vi "UHR-Fleezers Control (host) -Leonardo 04-2018 V2.vi"(0 "Tab Control":T5(tab)=enum."Trap Control (RF)") -> ()   [LabVIEW 2013] (continued)
        n954 = event-data() -> ()  [unwired: 7 out]
        n955 = call "hamilton_controller.vi"("Open?"="Inject Bottom", "valve"=enum16{"A", "B", "C", "D", "ALL"}."C", "action"=T21."MOVE VALVE") -> ()  [unwired: 8 in, 1 out]
      }
      event "Shunt:": Value Change {
        n956 = event-data() -> ()  [unwired: 7 out]
        n957 = call "hamilton_controller.vi"("Open?"="Shunt:", "valve"=enum16{"A", "B", "C", "D", "ALL"}."D", "action"=T21."MOVE VALVE") -> ()  [unwired: 8 in, 1 out]
      }
      event "Flip Green Filter": Value Change {
        n958 = event-data() -> ()  [unwired: 7 out]
        n959 = local write "Flip Green Filter"("Flip Green Filter") -> ()
        n960 = flat-sequence {
          tunnel: w1540 -> [w1545]
          tunnel: w1539 -> [w1544]
          tunnel: [w1542] -> w1537
          tunnel: [w1541] -> w1536
          tunnel: [w1547] -> w1535
          tunnel: w1537 -> [w1547]
          tunnel: [w1546] -> w1534
          tunnel: w1536 -> [w1546]
          tunnel: w1535 -> [w1551]
          tunnel: w1534 -> [w1550]
          tunnel: [w1549] -> w1538
          frame #0 {
            n961 = xnode "Read/Write Control"("FPGA VI Reference In"=w1545, "error in"=w1544, "Green Filter Flipper"=TRUE) -> ("FPGA VI Reference Out"=w1542:T20, "error out"=w1541:errorcluster)
          }
          frame #1 {
            n962 = Wait (ms)(milliseconds to wait=u32 100) -> ()  [unwired: 1 out]
          }
          frame #2 {
            n963 = xnode "Read/Write Control"("FPGA VI Reference In"=w1551, "error in"=w1550, "Green Filter Flipper"=FALSE) -> ("error out"=w1549:errorcluster)  [unwired: 1 out]
          }
        }
      }
      event "Pump 1 contents", "Pump 3 contents": Value Change {
        n964 = event-data() -> ()  [unwired: 7 out]
        n965 = local read "Pump 1 contents"() -> (→"Pump 1 cont disp":string)
        n966 = local read "Pump 3 contents"() -> (→"Pump 3 cont disp":string)
      }
      event "Reset Trap Pos. FB": Value Change {
        n967 = event-data() -> ()  [unwired: 7 out]
        n968 = xnode "Read/Write Control"("FPGA VI Reference In"=w1557, "error in"=w1556, "Trap Pos. FB Reset"="Reset Trap Pos. FB") -> ()  [unwired: 2 out]
      }
      event "Trap Pos. FB ON": Value Change {
        n969 = event-data() -> ()  [unwired: 7 out]
        n970 = xnode "Read/Write Control"("FPGA VI Reference In"=w1572, "error in"=w1571) -> ("FPGA VI Reference Out"=w1569:T20, "BD1 Frequency Out 1"=w1566:u64)  [unwired: 1 out]
        n971 = To Double Precision Float(number=w1566) -> (double precision float=w1565:dbl)
        n972 = Multiply(x=49125000.0, y=6.0) -> (x*y=w1564:dbl)
        n973 = Multiply(x=w1565, y=w1564) -> (x*y=w1562:dbl)
        n974 = Scale By Power Of 2(n=-48, x=w1562) -> (x*2^n=w1561:dbl)
        n975 = Divide(x=w1561, y=1000000.0) -> (x/y=w1558:dbl)
        n976 = flat-sequence {
          tunnel: [w1575] -> w1570
          tunnel: w1569 -> [w1576]
          tunnel: w1566 -> [w1574]
          tunnel: "Trap Pos. FB ON" -> [w1573]
          tunnel: "Trap Pos. FB ON" -> [w1582]
          tunnel: w1570 -> [w1581]
          tunnel: "Trap Pos. FB ON" -> [w1584]
          tunnel: w1558 -> [w1583]
          frame #0 {
            n977 = case shown="False" w1573 {
              tunnel: w1576 -> [w1579 w1580]
              tunnel: [w1578 w1580] -> w1575
              tunnel: w1574 -> [w1577 _]
              frame False {
                n978 = xnode "Read/Write Control"("FPGA VI Reference In"=w1579, "BD 1 Frequency 1"=w1577) -> ("FPGA VI Reference Out"=w1578:T20)  [unwired: 1 in, 1 out]
              }
              frame True {
              }
            }
          }
          frame #1 {
            n979 = xnode "Read/Write Control"("FPGA VI Reference In"=w1581, "Force feedback"=w1582) -> ()  [unwired: 1 in, 2 out]
          }
          frame #2 {
            n980 = case shown="False" w1584 {
              tunnel: w1583 -> [w1586 _]
              frame False {
                n981 = Subtract(x=90.0, y=w1586) -> (x-y=w1585:dbl)
                n982 = property on="Trap Delta (MHz)" class="DigNum (strict)"("Val(Sgnl)"=w1585) -> ()  [unwired: 2 in, 2 out]
              }
              frame True {
              }
            }
          }
        }
      }
      event "Diff. FB.", "Trap Pos. FB Gains", "Trap Pos. FB Mult Factor", "Trap Pos. FB Offset Factor", "Trap Pos FB Negate Action", "Trap Pos FB Monitor\nT1 or T2", "Negate Diff?": Value Change {
        n983 = event-data() -> ()  [unwired: 7 out]
        n984 = xnode "Read/Write Control"("FPGA VI Reference In"=w1598, "error in"=w1597, "Trap pos. FB Range"="Trap Pos. FB Range", "Trap Pos. FB Gains"="Trap Pos. FB Gains", "Trap Pos. FB Mult Factor"="Trap Pos. FB Mult Factor", "Trap Pos. FB Offset Factor"="Trap Pos. FB Offset Factor", "Trap Pos FB Negate Action"="Trap Pos FB Negate Action", "Trap Pos FB Monitor T1 or T2"="Trap Pos FB Monitor\nT1 or T2", "AI1 X Scale"="Trap Pos. AI1 X Pre-scale", "Negate Diff?"="Negate Diff?", "Diff FB Measurement?"="Diff. FB.") -> ()  [unwired: 2 out]
      }
      event "Trap Pos FB SP": Value Change {
        n985 = event-data() -> ()  [unwired: 7 out]
        n986 = xnode "Read/Write Control"("FPGA VI Reference In"=w1601, "error in"=w1600, "Trap Pos. FB SP"="Trap Pos FB SP") -> ()  [unwired: 2 out]
      }
      event "Simulate stepping": Value Change {
        n987 = event-data() -> ()  [unwired: 7 out]
        n988 = flat-sequence {
          tunnel: w1603 -> [w1606]
          tunnel: [w1605] -> _
          tunnel: w1602 -> [w1604]
          frame #0 {
            n989 = while {
              tunnel: w1606 -> [w1634]
              tunnel: [w1633] -> w1605 mode=indexing
              tunnel: w1604 -> [w1632]
              i -> [w1618]
              stop <- w1615 stop-if-true
              w1608 = 1000.0
              n990 = Divide(x="Backtrack probability", y=100) -> (x/y=w1642:dbl)
              n991 = Random Number (0-1)() -> (number: 0 to 1=w1643:dbl)
              n992 = Greater?(x=w1643, y=w1642) -> (0:w1641:bool)
              n993 = Select(t=1, s=w1641, f=-1) -> (s? t:f=w1638:i32)
              n994 = local read "BD 1 Frequency 2 (MHz)"() -> (w1613:dbl)
              n995 = Multiply(x=w1638, y="Step size (nm)") -> (x*y=w1636:dbl)
              "Step taken" <- w1636
              n996 = Divide(x=w1636, y=168.33) -> (x/y=w1611:dbl)
              n997 = local read "BD 1 Frequency 1 (MHz)"() -> (w1612:dbl)
              n998 = local read "X RF Frequency Limits (MHz)"() -> (w1631:T16)
              n999 = local read "Y RF Frequency Limits (MHz)"() -> (w1630:T16)
              n1000 = Subtract(x=w1612, y=w1611) -> (x-y=w1610:dbl)
              n1001 = local write "BD 1 Frequency 1 (MHz)"(w1610) -> ()
              n1002 = local read "BD 2 Frequency 1 (MHz)"() -> (w1628:dbl)
              n1003 = local read "BD 2 Frequency 2 (MHz)"() -> (w1629:dbl)
              n1004 = call "set RF board frequency - interlace.vi"("Board 2 Frequency Limits"=w1630, "Board 1 Frequency Limits"=w1631, "error in"=w1634, "FPGA VI Reference In"=w1632, "Board 2 Frequency 2 (MHz)"=w1629, "Board 2 Frequency 1 (MHz)"=w1628, "Board 1 Frequency 2 (MHz)"=w1613, "Board 1 Frequency 1  (MHz)"=w1610) -> ("error out"=w1633:errorcluster)  [unwired: 2 in, 1 out]
              n1005 = Subtract(x=w1613, y=w1610) -> (x-y=w1627:dbl)
              n1006 = Subtract(x=w1629, y=w1628) -> (x-y=w1626:dbl)
              n1007 = Square(x=w1626) -> (x^2=w1624:dbl)
              n1008 = Square(x=w1627) -> (x^2=w1625:dbl)
              n1009 = Add(x=w1625, y=w1624) -> (x+y=w1623:dbl)
              n1010 = Square Root(x=w1623) -> (sqrt(x)=w1614:dbl)
              n1011 = local write "Trap Delta (MHz)"(w1614) -> ()
              n1012 = property on="Initial delta (MHz)" class="DigNum (strict)"("Val(Sgnl)"=w1614) -> ()  [unwired: 2 in, 2 out]
              n1013 = Multiply(x="Mean dwell time (s)", y=w1608) -> (x*y=w1620:dbl)
              n1014 = case shown="\"Gamma2\"" "Distribution" {
                tunnel: w1620 -> [w1647 w1651 w1654]
                tunnel: [w1647 w1648 w1655] -> w1609
                frame "uniform", Default {
                }
                frame "Exponential" {
                  n1015 = call-poly <vilib>:"Continuous Random.vi"("b"=w1651, "samples"=1) -> ("exp random data"=w1649:dbl[])  [unwired: 8 in, 1 out]
                  n1016 = Index Array(array=w1649) -> (element=w1648:dbl)  [unwired: 1 in]
                }
                frame "Gamma2" {
                  w1652 = 2.0
                  # "Note: the shape and scale\nparameters of the gamma\nare inverted because LabView..."
                  n1017 = Divide(x=w1654, y=w1652) -> (x/y=w1653:dbl)
                  n1018 = call-poly <vilib>:"Continuous Random.vi"("c"=w1653, "b"=w1652, "samples"=1) -> ("gamma random numbers"=w1656:dbl[])  [unwired: 7 in, 1 out]
                  n1019 = Index Array(array=w1656) -> (element=w1655:dbl)  [unwired: 1 in]
                }
              }
              n1020 = Divide(x=w1609, y=w1608) -> (x/y=→"Step duration":dbl)
              n1021 = To Unsigned Long Integer(number=w1609) -> (unsigned 32bit integer=w1621:u32)
              n1022 = Add(x=w1618, y=1) -> (x+y=w1617:i32)
              n1023 = Wait (ms)(milliseconds to wait=w1621) -> ()  [unwired: 1 out]
              n1024 = Equal?(x=w1617, y="Number of steps") -> (x = y?=w1615:bool)
            }
          }
          frame #1 {
            n1025 = local write "Simulate stepping"(FALSE) -> ()
          }
        }
      }
      event "Set SP to Reading": Value Change {
        n1026 = event-data() -> ()  [unwired: 7 out]
        n1027 = local read "Trap Pos FB Monitor\nT1 or T2"() -> (w1666:bool)
        n1028 = local read "Trap X AI1 (DMA)"() -> (w1669:T13)
        n1029 = local read "Trap X (AI1)"() -> (w1672:T1)
        n1030 = Unbundle By Name(w1672) -> ("Trap 1"=w1671:fxp<+/-,16,1>, "Trap 2"=w1670:fxp<+/-,16,1>)
        n1031 = Unbundle By Name(w1669) -> ("Set 1"=w1668:fxp<+/-,16,1>, "Set 2"=w1667:fxp<+/-,16,1>)
        n1032 = Select(t=w1671, s=w1666, f=w1670) -> (s? t:f=w1665:fxp<+/-,16,1>)
        n1033 = Select(t=w1668, s=w1666, f=w1667) -> (s? t:f=w1664:fxp<+/-,16,1>)
        n1034 = Not(x="Set SP Using...") -> (.not. x?=w1659:bool)
        n1035 = Select(t=w1665, s=w1659, f=w1664) -> (s? t:f=w1660:fxp<+/-,16,1>)
        n1036 = xnode "Read/Write Control"("FPGA VI Reference In"=w1662, "error in"=w1661, "Trap Pos. FB SP"=w1660) -> ()  [unwired: 2 out]
        n1037 = local write "Trap Pos FB SP"(w1660) -> ()
      }
      event "Trap Pos. FB Out Scale 2^n": Value Change {
        n1038 = event-data() -> ()  [unwired: 7 out]
        n1039 = Scale By Power Of 2(n="Trap Pos. FB Out Scale 2^n", x=ext 1.0) -> (x*2^n=w1674:ext)
        n1040 = property on="Trap Pos. FB Mult Factor" class="DigNum (strict)"("Val(Sgnl)"=w1674) -> ()  [unwired: 2 in, 2 out]
      }
      event "Trap Pos FB Int Count": Value Change {
        n1041 = event-data() -> ()  [unwired: 7 out]
        n1042 = xnode "Read/Write Control"("FPGA VI Reference In"=w1679, "error in"=w1678, "Trap Pos FB Int Count"="Trap Pos FB Int Count") -> ()  [unwired: 2 out]
      }
      event "Target Force (pN)", "Setpoint offset\nCorrection values", "Raster target force (pN)": Value Change {
        w1687 = 2.0
        n1043 = event-data() -> ()  [unwired: 7 out]
        n1044 = local read "B factor"() -> (w1718:dbl)
        n1045 = To Fixed-Point(number=w1718) -> (fixed-point=w1717:fxp<+/-,16,16>)  [unwired: 1 in]
        n1046 = xnode "Read/Write Control"("FPGA VI Reference In"=w1681, "B factor"=w1717) -> ("BD1 Frequency Out 1"=w1708:u64)  [unwired: 1 in, 2 out]
        n1047 = local read "BD 1 Frequency 2 (MHz)"() -> (w1707:dbl)
        n1048 = local read "Target Force (pN)"() -> (w1693:dbl)
        n1049 = To Double Precision Float(number=w1708) -> (double precision float=w1714:dbl)
        n1050 = Multiply(x=49125000.0, y=6.0) -> (x*y=w1713:dbl)
        n1051 = Multiply(x=w1714, y=w1713) -> (x*y=w1711:dbl)
        n1052 = Scale By Power Of 2(n=-48, x=w1711) -> (x*2^n=w1710:dbl)
        n1053 = Divide(x=w1710, y=1000000.0) -> (x/y=w1706:dbl)
        n1054 = Subtract(x=w1707, y=w1706) -> (x-y=w1705:dbl)
        n1055 = local read "T1 kappa_x (pN/nm)"() -> (w1694:dbl)
        n1056 = local read "T1 alpha_x (nm/V)"() -> (w1695:dbl)
        n1057 = local read "Negate offset difference"() -> (w1696:bool)
        n1058 = local read "Offset file step size"() -> (w1704:dbl)
        n1059 = Multiply(x="Raster target force (pN)", y=w1687) -> (x*y=w1686:dbl)
        n1060 = Multiply(x=w1693, y=w1687) -> (x*y=w1692:dbl)
        n1061 = local read "Setpoint offset\nCorrection values"() -> (w1701:dbl[])
        n1062 = Divide(x=w1705, y=w1704) -> (x/y=w1703:dbl)
        n1063 = Select(t=-1, s=w1696, f=1) -> (s? t:f=w1697:i32)
        n1064 = To Long Integer(number=w1703) -> (32bit integer=w1702:i32)
        n1065 = Multiply(x=w1695, y=w1694) -> (x*y=w1685:dbl)
        n1066 = Divide(x=w1692, y=w1685) -> (x/y=w1691:dbl)
        n1067 = Index Array(array=w1701, index=w1702) -> (element=w1700:dbl)
        n1068 = Divide(x=w1686, y=w1685) -> (x/y=w1684:dbl)
        n1069 = Multiply(x=w1697, y=w1700) -> (x*y=w1683:dbl)
        n1070 = Add(x=w1691, y=w1683) -> (x+y=w1690:dbl)
        n1071 = Add(x=w1684, y=w1683) -> (x+y=w1682:dbl)
        n1072 = To Fixed-Point(number=w1682) -> (fixed-point=w1680:fxp<+/-,16,1>)  [unwired: 1 in]
        n1073 = To Fixed-Point(number=w1690) -> (fixed-point=w1689:fxp<+/-,16,1>)  [unwired: 1 in]
        n1074 = property on="Trap Pos FB SP" class="DigNum (strict)"("Val(Sgnl)"=w1689) -> ()  [unwired: 2 in, 2 out]
        n1075 = xnode "Read/Write Control"("FPGA VI Reference In"=w1681, "Raster setpoint"=w1680) -> ()  [unwired: 1 in, 2 out]
      }
      event "Read setpoint correction\nfile": Value Change {
        n1076 = event-data() -> ()  [unwired: 7 out]
        n1077 = local write "Read setpoint correction\nfile"(FALSE) -> ()
        n1078 = Open/Create/Replace File(file path (use dialog)="Setpoint correction\noffset file", operation (0:open)=T24."open", access (0:read/write)=enum16{"read/write", "read-only", "write-only"}."read-only") -> (refnum out=w1743:refnum<file>)  [unwired: 1 in, 4 out]
        n1079 = Deny Access(7:w1743) -> (3:w1741:refnum<file>)  [unwired: 1 in, 2 out]
        n1080 = Read from Binary File(5:0.0, 9:T30."big-endian, network order" ("byte order (0:big-endian, network order)"), 10:-1 ("count (1)"), 11:w1741) -> (2:w1734:dbl[], 3:w1740:refnum<file>)  [unwired: 1 in, 3 out]
        n1081 = Close File(refnum=w1740) -> ()  [unwired: 1 in, 2 out]
        n1082 = Index Array(array=w1734, index=0) -> (element=w1730:dbl)
        n1083 = local write "Offset file step size"(w1730) -> ()
        n1084 = Array Subset(array=w1734, index=3) -> (w1733:dbl[])  [unwired: 1 in]
        n1085 = local read "T1 kappa_x (pN/nm)"() -> (w1728:dbl)
        n1086 = local read "T1 alpha_x (nm/V)"() -> (w1729:dbl)
        n1087 = local read "T2 alpha_x (nm/V)"() -> (w1727:dbl)
        n1088 = local read "T2 kappa_x (pN/nm)"() -> (w1726:dbl)
        n1089 = Decimate 1D Array(w1733) -> (w1721:dbl[], w1722:dbl[])  [unwired: 1 out]
        n1090 = local read "Offset Values"() -> (w1732:T14)
        n1091 = Multiply(x=w1729, y=w1728) -> (x*y=w1724:dbl)
        n1092 = Multiply(x=w1727, y=w1726) -> (x*y=w1725:dbl)
        n1093 = Bundle By Name(cluster=w1732, "Trap 1X offset"=w1721, "Trap 2X offset"=w1722) -> (w1731:T14)
        n1094 = Divide(x=w1725, y=w1724) -> (x/y=w1723:dbl)
        n1095 = property on="B factor" class="DigNum (strict)"("Val(Sgnl)"=w1723) -> ()  [unwired: 2 in, 2 out]
        n1096 = Multiply(x=w1722, y=w1723) -> (x*y=w1720:dbl[])
        n1097 = local write "Offset Values"(w1731) -> ()
        n1098 = Subtract(x=w1721, y=w1720) -> (x-y=w1719:dbl[])
        n1099 = property on="Setpoint offset\nCorrection values" class="Arr (strict)"("Val(Sgnl)"=w1719) -> ()  [unwired: 2 in, 2 out]
      }
      event "MCL Tracking": Value Change {
        n1100 = event-data() -> ()  [unwired: 7 out]
        n1101 = case shown="True" "MCL Tracking" {
          frame False {
            n1102 = local read "Current MCL (V)"() -> (w1748:dbl)
            n1103 = local write "AO2"(w1748) -> ()
          }
          frame True {
            n1104 = local read "BD 1 Frequency 1 (MHz)"() -> (→"Zero T1 position":dbl)
            n1105 = local read "AO2"() -> (→"Zero MCL x position":dbl)
          }
        }
      }
    }
    "error out 2" <- w762
    n1106 = node-c288() -> ()  [unwired: 1 in, 1 out]
  }
  n1107 = timed-loop "Run Scripts, including: stage motion" {
    timing: w97 -> [_]
    timing-out: [_] -> w96
    tunnel: w55 -> [_]
    stop <- w1752 stop-if-true
    n1108 = node-c288() -> ()  [unwired: 1 in, 1 out]
    n1109 = event shown="[5] \"Profile\": Value Change" {
      selector: _ -> [_ _ _ _ _ _ _ _ _ _ _ _]
      dyn-events: _ -> [_ _ _ _ _ _ _ _ _ _ _ _]
      timeout: 50 -> [_ _ _ _ _ _ _ _ _ _ _ _]
      tunnel: ["Move Cap. 1 (DNA Top)" _ "Cal/Data Acq. Spot" "Dump Beads" "Dip for Protein" _ "Got ADig bead" "Got DNA bead" "Take Stepping Data" _ "Take Detection Laser\nImage" _] -> _
      tunnel: [_ _ _ _ _ _ _ _ _ _ _ w1960] -> w1752
      event "Move Cap. 1 (DNA Top)": Value Change {
        n1110 = event-data() -> ()  [unwired: 1 in, 5 out]
        n1111 = local write "Move Cap. 1 (DNA Top)"(FALSE ("Move Cap. 1 (DNA Right)")) -> ()
        n1112 = flat-sequence {
          tunnel: "Cap 1 Samp Flow ON" -> [w1758]
          frame #0 {
            n1113 = local write "Stage Moving"(FALSE ("Stage Moving")) -> ()
            n1114 = case "stop flow" shown="True" w1758 {
              frame False {
              }
              frame True {
                n1115 = call "hamilton_controller.vi"("Open?"=FALSE, "valve"=enum16{"A", "B", "C", "D", "ALL"}."C", "action"=T21."MOVE VALVE") -> ()  [unwired: 8 in, 1 out]
              }
            }
            n1116 = case shown="True" TRUE {
              tunnel: "Cap 1 T ON" -> [w1767 w1768]
              frame False {
                n1117 = property on="Trap 1 (ON/OFF)" class="Bool (strict)"("Val(Sgnl)"=w1767) -> ()  [unwired: 2 in, 2 out]
              }
              frame True {
                n1118 = property on="Trap 2 (ON/OFF)" class="Bool (strict)"("Val(Sgnl)"=w1768) -> ()  [unwired: 2 in, 2 out]
              }
            }
            n1119 = call <vilib>:"Beep.vi"() -> ()  [unwired: 3 in, 9 out]
            n1120 = case shown="True" "Cap 1 Flow ON" {
              frame False {
              }
              frame True {
                n1121 = property on="Main:" class="Bool (strict)"("Val(Sgnl)"=TRUE ("Value (Signaling)")) -> ()  [unwired: 2 in, 2 out]
              }
            }
          }
        }
      }
      event Timeout {
        n1122 = event-data() -> ()  [unwired: 1 in, 2 out]
      }
      event "Cal/Data Acq. Spot": Value Change {
        # "wait for calibration file\nto be written"
        # "signal save cal true\nthis tells the data \nacquisition loop to\nstart sending the data\nto a calibration file"
        # "separate traps to\nthe desired trap delta"
        # "move stage to data acquisition spot"
        # "CHANGE FISH FOR TETHER BACK\nTO TRUE VALUE HERE."
        n1123 = event-data() -> ()  [unwired: 1 in, 5 out]
        n1124 = local write "Cal/Data Acq. Spot"(FALSE ("Cal/Data Acq. Spot")) -> ()
        n1125 = flat-sequence {
          tunnel: ["Cal @ (MHz)"] -> w1769
          tunnel: w1769 -> [w1779]
          tunnel: w1769 -> [w1800]
          frame #0 {
            n1126 = property on="Trap Delta (MHz)" class="DigNum (strict)"("Val(Sgnl)"="Cal @ (MHz)") -> ()  [unwired: 2 in, 2 out]
            n1127 = call <vilib>:"Beep.vi"() -> ()  [unwired: 3 in, 9 out]
          }
          frame #1 {
            n1128 = Wait (ms)(milliseconds to wait=u32 100) -> ()  [unwired: 1 out]
          }
          frame #2 {
            n1129 = property on="Save Calibration" class="Bool (strict)"("Val(Sgnl)"=TRUE ("Value (Signaling)")) -> ()  [unwired: 2 in, 2 out]
          }
          frame #3 {
            n1130 = Wait (ms)(milliseconds to wait=u32 4000) -> ()  [unwired: 1 out]
          }
          frame #4 {
            n1131 = while {
              stop <- w1776 stop-if-true
              n1132 = local read "Saving..."() -> (w1777:bool)
              n1133 = Wait (ms)(milliseconds to wait=u32 100) -> ()  [unwired: 1 out]
              n1134 = Not(x=w1777) -> (.not. x?=w1776:bool)
            }
          }
          frame #5 {
            n1135 = case shown="True" "W/ Offset 1" {
              tunnel: w1779 -> [_ w1781]
              frame False {
              }
              frame True {
                n1136 = stacked-sequence {
                  tunnel: w1781 -> [_ _ _ _ _ _ _ w1798]
                  frame #0 {
                    n1137 = Replace Array Subset(array=u32[] [0] ("Index Values"), new element="Offset 1 Set", index=0) -> (w1782:u32[])
                    n1138 = property on="Saved AOD Raster Scan Parameter Sets" class="Arr (strict)"("Index Values"=w1782) -> ()  [unwired: 2 in, 2 out]
                    n1139 = property on="Trap Delta (MHz)" class="DigNum (strict)"("Val(Sgnl)"="Offset 1 Start (MHz)") -> ()  [unwired: 2 in, 2 out]
                  }
                  frame #1 {
                    n1140 = Wait (ms)(milliseconds to wait=u32 200) -> ()  [unwired: 1 out]
                  }
                  frame #2 {
                    n1141 = property on="Load parameters" class="Bool (strict)"("Val(Sgnl)"=TRUE ("Value (Signaling)")) -> ()  [unwired: 2 in, 2 out]
                  }
                  frame #3 {
                    n1142 = Wait (ms)(milliseconds to wait=u32 200) -> ()  [unwired: 1 out]
                  }
                  frame #4 {
                    n1143 = property on="Trap Raster Scan" class="Bool (strict)"("Val(Sgnl)"=TRUE ("Value (Signaling)")) -> ()  [unwired: 2 in, 2 out]
                  }
                  frame #5 {
                    n1144 = Wait (ms)(milliseconds to wait=u32 2000) -> ()  [unwired: 1 out]
                  }
                  frame #6 {
                    n1145 = while {
                      stop <- w1795 stop-if-true
                      n1146 = local read "Raster Scanning..."() -> (w1797:bool)
                      n1147 = local read "Saving..."() -> (w1793:bool)
                      n1148 = Wait (ms)(milliseconds to wait=u32 100) -> ()  [unwired: 1 out]
                      n1149 = Not(x=w1793) -> (.not. x?=w1792:bool)
                      n1150 = Not(x=w1797) -> (.not. x?=w1794:bool)
                      n1151 = And(x=w1794, y=w1792) -> (x .and. y?=w1795:bool)
                    }
                  }
                  frame #7 {
                    n1152 = property on="Trap Delta (MHz)" class="DigNum (strict)"("Val(Sgnl)"=w1798) -> ()  [unwired: 2 in, 2 out]
                  }
                }
              }
            }
          }
          frame #6 {
            n1153 = local read "Save ave N"() -> (w1799:dbl)
            n1154 = case shown="True" "W/ Offset 2" {
              tunnel: w1800 -> [_ w1806]
              tunnel: w1799 -> [_ w1805]
              frame False {
                n1155 = Multiply(x="Cal read wait (s)", y=u32 1000 ("milliseconds to wait")) -> (x*y=w1803:u32)
                n1156 = Wait (ms)(milliseconds to wait=w1803) -> ()  [unwired: 1 out]
              }
              frame True {
                n1157 = stacked-sequence {
                  tunnel: w1806 -> [_ _ _ _ _ _ _ _ _ w1827 _ _]
                  tunnel: w1805 -> [_ _ _ _ _ _ _ _ _ w1825 _ _]
                  frame #0 {
                    n1158 = property on="Save ave N" class="DigNum (strict)"("Val(Sgnl)"=1.0 ("Value (Signaling)")) -> ()  [unwired: 2 in, 2 out]
                  }
                  frame #1 {
                    n1159 = Wait (ms)(milliseconds to wait=u32 500) -> ()  [unwired: 1 out]
                  }
                  frame #2 {
                    n1160 = property on="Trap Delta (MHz)" class="DigNum (strict)"("Val(Sgnl)"="Offset 2 Start (MHz)") -> ()  [unwired: 2 in, 2 out]
                    n1161 = Replace Array Subset(array=u32[] [0] ("Index Values"), new element="Offset 2 Set", index=0) -> (w1811:u32[])
                    n1162 = property on="Saved AOD Raster Scan Parameter Sets" class="Arr (strict)"("Index Values"=w1811) -> ()  [unwired: 2 in, 2 out]
                  }
                  frame #3 {
                    n1163 = Wait (ms)(milliseconds to wait=u32 500) -> ()  [unwired: 1 out]
                  }
                  frame #4 {
                    n1164 = property on="Load parameters" class="Bool (strict)"("Val(Sgnl)"=TRUE ("Value (Signaling)")) -> ()  [unwired: 2 in, 2 out]
                  }
                  frame #5 {
                    n1165 = Wait (ms)(milliseconds to wait=u32 500) -> ()  [unwired: 1 out]
                  }
                  frame #6 {
                    n1166 = property on="Trap Raster Scan" class="Bool (strict)"("Val(Sgnl)"=TRUE ("Value (Signaling)")) -> ()  [unwired: 2 in, 2 out]
                  }
                  frame #7 {
                    n1167 = Wait (ms)(milliseconds to wait=u32 2000) -> ()  [unwired: 1 out]
                  }
                  frame #8 {
                    n1168 = while {
                      stop <- w1820 stop-if-true
                      n1169 = local read "Raster Scanning..."() -> (w1823:bool)
                      n1170 = local read "Saving..."() -> (w1821:bool)
                      n1171 = Wait (ms)(milliseconds to wait=u32 100) -> ()  [unwired: 1 out]
                      n1172 = Not(x=w1821) -> (.not. x?=w1819:bool)
                      n1173 = Not(x=w1823) -> (.not. x?=w1822:bool)
                      n1174 = And(x=w1822, y=w1819) -> (x .and. y?=w1820:bool)
                    }
                  }
                  frame #9 {
                    n1175 = property on="Trap Delta (MHz)" class="DigNum (strict)"("Val(Sgnl)"=w1827) -> ()  [unwired: 2 in, 2 out]
                    n1176 = property on="Saved AOD Raster Scan Parameter Sets" class="Arr (strict)"("Index Values"=u32[] [0]) -> ()  [unwired: 2 in, 2 out]
                    n1177 = property on="Save ave N" class="DigNum (strict)"("Val(Sgnl)"=w1825) -> ()  [unwired: 2 in, 2 out]
                  }
                  frame #10 {
                    n1178 = Wait (ms)(milliseconds to wait=u32 500) -> ()  [unwired: 1 out]
                  }
                  frame #11 {
                    n1179 = property on="Load parameters" class="Bool (strict)"("Val(Sgnl)"=TRUE ("Value (Signaling)")) -> ()  [unwired: 2 in, 2 out]
                  }
                }
              }
            }
          }
          frame #7 {
            n1180 = property on="Read Cal" class="Bool (strict)"("Val(Sgnl)"=TRUE ("Value (Signaling)")) -> ()  [unwired: 2 in, 2 out]
          }
          frame #8 {
            n1181 = Wait (ms)(milliseconds to wait=u32 500) -> ()  [unwired: 1 out]
          }
          frame #9 {
            n1182 = property on="Fish for Tether" class="Bool (strict)"("Val(Sgnl)"=FALSE ("Value (Signaling)")) -> ()  [unwired: 2 in, 2 out]
          }
        }
      }
      event "Dump Beads": Value Change {
        # "SCRIPT TO REMOVE BOTH BEADS FROM THE TRAPS. TURNS ON LIGHT WHICH INDICATES THAT STAGE IS MOVING. THEN STOPS SAVING DATA. \nSETS Sample Channel Flow TO TRUE. STOPS INTERLACING GREEN FLUORESCENCE. TURNS OFF Tether INDICATOR BECAUSE WE ARE THROWING IT\nAWAY. SHUTS OFF TRAP POSITION FEEDBACK."
        n1183 = event-data() -> ()  [unwired: 1 in, 5 out]
        n1184 = flat-sequence {
          frame #0 {
            w1834 = FALSE ("Fl. Triggered...")
            w1835 = TRUE ("Stage Moving")
            n1185 = local read "Saving..."() -> (w1836:bool)
            n1186 = local write "Fl. Triggered..."(w1834) -> ()
            n1187 = local write "Stage Moving"(w1835) -> ()
            n1188 = local write "Tether"(w1834) -> ()
            n1189 = property on="Green Laser ON/Interlacing" class="Bool (strict)"("Val(Sgnl)"=w1834) -> ()  [unwired: 2 in, 2 out]
            n1190 = property on="Trap Pos. FB ON" class="Bool (strict)"("Val(Sgnl)"=w1834) -> ()  [unwired: 2 in, 2 out]
            n1191 = property on="Inject Bottom" class="Bool (strict)"("Val(Sgnl)"=w1835) -> ()  [unwired: 2 in, 2 out]
            n1192 = local write "Stop Saving"(w1836) -> ()
          }
          frame #1 {
            w1837 = FALSE ("Value (Signaling)")
            # "TURNS TRAPS OFF SO THAT\nBEADS REMAIN AT DUMP \nBEADS POSITION"
            n1193 = property on="Trap 1 (ON/OFF)" class="Bool (strict)"("Val(Sgnl)"=w1837) -> ()  [unwired: 2 in, 2 out]
            n1194 = property on="Trap 2 (ON/OFF)" class="Bool (strict)"("Val(Sgnl)"=w1837) -> ()  [unwired: 2 in, 2 out]
            n1195 = call <vilib>:"Beep.vi"() -> ()  [unwired: 3 in, 9 out]
          }
          frame #2 {
            n1196 = property on="Goto Bottom (F7)" class="Bool (strict)"("Val(Sgnl)"=TRUE ("Value (Signaling)")) -> ()  [unwired: 2 in, 2 out]
          }
          frame #3 {
            n1197 = Wait (ms)(milliseconds to wait=u32 8000) -> ()  [unwired: 1 out]
          }
          frame #4 {
            n1198 = property on="Trap Delta (MHz)" class="DigNum (strict)"("Val(Sgnl)"=20.0 ("Value (Signaling)")) -> ()  [unwired: 2 in, 2 out]
          }
          frame #5 {
            n1199 = property on="Trap 2 (ON/OFF)" class="Bool (strict)"("Val(Sgnl)"=TRUE ("Value (Signaling)")) -> ()  [unwired: 2 in, 2 out]
          }
          frame #6 {
            n1200 = property on="Inject Bottom" class="Bool (strict)"("Val(Sgnl)"=FALSE ("Value (Signaling)")) -> ()  [unwired: 2 in, 2 out]
          }
        }
      }
      event "Dip for Protein": Value Change {
        n1201 = event-data() -> ()  [unwired: 1 in, 5 out]
        n1202 = flat-sequence {
          frame #0 {
            n1203 = case shown="True" "Move Trap Before?" {
              frame False {
              }
              frame True {
                n1204 = property on="Trap Delta (MHz)" class="DigNum (strict)"("Val(Sgnl)"="Dip Trap Delta 1 (MHz)") -> ()  [unwired: 2 in, 2 out]
              }
            }
          }
          frame #1 {
            n1205 = Multiply(x="Duration (s)", y=1000.0) -> (x*y=w1846:dbl)
            n1206 = Wait (ms)(milliseconds to wait=w1846) -> ()  [unwired: 1 out]
          }
          frame #2 {
            n1207 = case shown="True" "Move Trap After?" {
              frame False {
              }
              frame True {
                n1208 = property on="Trap Delta (MHz)" class="DigNum (strict)"("Val(Sgnl)"="Dip Trap Delta 2 (MHz)") -> ()  [unwired: 2 in, 2 out]
              }
            }
          }
          frame #3 {
            n1209 = case shown="True" "Green ON After?" {
              frame False {
              }
              frame True {
                n1210 = property on="Green Laser ON/Interlacing" class="Bool (strict)"("Val(Sgnl)"=TRUE ("Value (Signaling)")) -> ()  [unwired: 2 in, 2 out]
              }
            }
          }
          frame #4 {
            n1211 = Wait (ms)(milliseconds to wait=u32 500) -> ()  [unwired: 1 out]
          }
          frame #5 {
            n1212 = case shown="True" "Save Data After?" {
              frame False {
              }
              frame True {
                n1213 = property on="Start Saving" class="Bool (strict)"("Val(Sgnl)"=TRUE ("Value (Signaling)")) -> ()  [unwired: 2 in, 2 out]
              }
            }
          }
        }
      }
      event "Profile": Value Change {
        n1214 = event-data() -> ()  [unwired: 1 in, 5 out]
        n1215 = flat-sequence {
          frame #0 {
            w1856 = 0.0 ("element")
            n1216 = Build Array(w1856, "Y change (mm)", w1856) -> ()  [unwired: 1 out]
          }
          frame #1 {
            # "stop saving"
            n1217 = local write "Stop Saving"(TRUE ("Stop Saving")) -> ()
            n1218 = local write "Stage Moving"(FALSE ("Stage Moving")) -> ()
          }
        }
      }
      event "Got ADig bead": Value Change {
        n1219 = event-data() -> ()  [unwired: 1 in, 5 out]
        n1220 = property on="Move Cap. 1 (DNA Top)" class="Bool (strict)"("Val(Sgnl)"=TRUE ("Value (Signaling)")) -> ()  [unwired: 2 in, 2 out]
        n1221 = property on="Inject Top:" class="Bool (strict)"("Val(Sgnl)"=FALSE ("Value (Signaling)")) -> ()  [unwired: 2 in, 2 out]
      }
      event "Got DNA bead": Value Change {
        n1222 = event-data() -> ()  [unwired: 1 in, 5 out]
        n1223 = property on="Cal/Data Acq. Spot" class="Bool (strict)"("Val(Sgnl)"=TRUE ("Value (Signaling)")) -> ()  [unwired: 2 in, 2 out]
        n1224 = property on="Main:" class="Bool (strict)"("Val(Sgnl)"=FALSE ("Value (Signaling)")) -> ()  [unwired: 2 in, 2 out]
      }
      event "Take Stepping Data": Value Change {
        n1225 = event-data() -> ()  [unwired: 1 in, 5 out]
        n1226 = local read "Save ave N"() -> (w1874:dbl)
        n1227 = flat-sequence {
          tunnel: w1874 -> [w1876]
          tunnel: [w1876] -> w1869
          tunnel: [w1878] -> w1870
          tunnel: w1869 -> [w1878]
          tunnel: [w1880] -> w1871
          tunnel: w1870 -> [w1880]
          tunnel: [w1883] -> w1872
          tunnel: w1871 -> [w1883]
          tunnel: [w1885] -> w1873
          tunnel: w1872 -> [w1885]
          tunnel: [w1887] -> w1867
          tunnel: w1873 -> [w1887]
          tunnel: w1867 -> [w1890]
          tunnel: [w1890] -> w1866
          tunnel: w1866 -> [w1891]
          tunnel: [w1891] -> w1868
          tunnel: w1868 -> [w1897]
          frame #0 {
            n1228 = property on="Save ave N" class="DigNum (strict)"("Val(Sgnl)"="Save ave factor") -> ()  [unwired: 2 in, 2 out]
          }
          frame #1 {
            n1229 = Wait (ms)(milliseconds to wait=u32 100) -> ()  [unwired: 1 out]
          }
          frame #2 {
            n1230 = local read "Offset 2 Start (MHz)"() -> (w1882:dbl)
            n1231 = property on="Saved AOD Raster Scan Parameter Sets" class="Arr (strict)"("Index Values"=u32[] [2]) -> ()  [unwired: 2 in, 2 out]
            n1232 = property on="Trap Delta (MHz)" class="DigNum (strict)"("Val(Sgnl)"=w1882) -> ()  [unwired: 2 in, 2 out]
          }
          frame #3 {
            n1233 = property on="Load parameters" class="Bool (strict)"("Val(Sgnl)"=TRUE ("Value (Signaling)")) -> ()  [unwired: 2 in, 2 out]
          }
          frame #4 {
            n1234 = Wait (ms)(milliseconds to wait=u32 100) -> ()  [unwired: 1 out]
          }
          frame #5 {
            n1235 = property on="Trap Raster Scan" class="Bool (strict)"("Val(Sgnl)"=TRUE ("Value (Signaling)")) -> ()  [unwired: 2 in, 2 out]
          }
          frame #6 {
            n1236 = Wait (ms)(milliseconds to wait=u32 1000) -> ()  [unwired: 1 out]
          }
          frame #7 {
            n1237 = while {
              stop <- w1894 stop-if-true
              n1238 = local read "Raster Scanning..."() -> (w1896:bool)
              n1239 = local read "Saving..."() -> (w1895:bool)
              n1240 = Not(x=w1895) -> (.not. x?=w1892:bool)
              n1241 = Not(x=w1896) -> (.not. x?=w1893:bool)
              n1242 = And(x=w1893, y=w1892) -> (x .and. y?=w1894:bool)
            }
          }
          frame #8 {
            n1243 = property on="Save ave N" class="DigNum (strict)"("Val(Sgnl)"=w1897) -> ()  [unwired: 2 in, 2 out]
          }
        }
      }
      event "Step Size (nm)": Value Change {
        n1244 = event-data() -> ()  [unwired: 1 in, 5 out]
        n1245 = flat-sequence {
          frame #0 {
            n1246 = property on="Saved AOD Raster Scan Parameter Sets" class="Arr (strict)"("Index Values"=u32[] [1]) -> ()  [unwired: 2 in, 2 out]
          }
          frame #1 {
            n1247 = Multiply(x="N Steps", y="Step Size (nm)") -> (x*y=w1899:dbl)
            n1248 = property on="Scan Speed AOD (nm/s) 2" class="DigNum (strict)"("Value"="Step Size (nm)") -> ()  [unwired: 2 in, 2 out]
            n1249 = property on="Step Size AOD (nm) 2" class="DigNum (strict)"("Value"="Step Size (nm)") -> ()  [unwired: 2 in, 2 out]
            n1250 = property on="Scan Range AOD (nm) 2" class="DigNum (strict)"("Value"=w1899) -> ()  [unwired: 2 in, 2 out]
          }
        }
      }
      event "Take Detection Laser\nImage": Value Change {
        n1251 = event-data() -> ()  [unwired: 1 in, 5 out]
        n1252 = flat-sequence {
          tunnel: [w1927] -> w1917
          tunnel: [w1926] -> w1910
          tunnel: [w1925] -> w1902
          tunnel: [w1930] -> w1918
          tunnel: w1917 -> [w1930]
          tunnel: [w1929] -> w1911
          tunnel: w1910 -> [w1929]
          tunnel: [w1928] -> w1903
          tunnel: w1902 -> [w1928]
          tunnel: [w1934] -> w1919
          tunnel: w1918 -> [w1934]
          tunnel: [w1933] -> w1912
          tunnel: w1911 -> [w1933]
          tunnel: [w1932] -> w1904
          tunnel: w1903 -> [w1932]
          tunnel: [w1940] -> w1920
          tunnel: w1919 -> [w1940]
          tunnel: [w1939] -> w1913
          tunnel: w1912 -> [w1939]
          tunnel: [w1938] -> w1905
          tunnel: w1904 -> [w1938]
          tunnel: [w1944] -> w1921
          tunnel: w1920 -> [w1944]
          tunnel: [w1943] -> w1914
          tunnel: w1913 -> [w1943]
          tunnel: [w1942] -> w1906
          tunnel: w1905 -> [w1942]
          tunnel: [w1948] -> w1922
          tunnel: w1921 -> [w1948]
          tunnel: [w1947] -> w1915
          tunnel: w1914 -> [w1947]
          tunnel: [w1946] -> w1907
          tunnel: w1906 -> [w1946]
          tunnel: [w1952] -> w1923
          tunnel: w1922 -> [w1952]
          tunnel: [w1951] -> w1916
          tunnel: w1915 -> [w1951]
          tunnel: [w1950] -> w1908
          tunnel: w1907 -> [w1950]
          tunnel: w1923 -> [w1958]
          tunnel: w1916 -> [w1957]
          tunnel: [w1955] -> w1909
          tunnel: w1908 -> [w1955]
          tunnel: w1909 -> [w1959]
          frame #0 {
            n1253 = local read "Green Laser ON/Interlacing"() -> (w1927:bool)
            n1254 = local read "Green laser mode"() -> (w1926:enum32{"Laser ON", "Laser OFF", "Interlace"})
            n1255 = local read "Green FB On/Off"() -> (w1925:bool)
          }
          frame #1 {
            n1256 = property on="Green FB On/Off" class="Bool (strict)"("Val(Sgnl)"=FALSE ("Value (Signaling)")) -> ()  [unwired: 2 in, 2 out]
          }
          frame #2 {
            n1257 = property on="Green Laser ON/Interlacing" class="Bool (strict)"("Val(Sgnl)"=TRUE ("Value (Signaling)")) -> ()  [unwired: 2 in, 2 out]
            n1258 = property on="Flip Green Filter" class="Bool (strict)"("Val(Sgnl)"=TRUE ("Value (Signaling)")) -> ()  [unwired: 2 in, 2 out]
            n1259 = property on="Green laser mode" class="RadioBtnsControl (strict)"("Val(Sgnl)"=enum32{"Laser ON", "Laser OFF", "Interlace"}."Laser ON" ("Value (Signaling)")) -> ()  [unwired: 2 in, 2 out]
          }
          frame #3 {
            n1260 = Wait (ms)(milliseconds to wait=u32 500) -> ()  [unwired: 1 out]
          }
          frame #4 {
            n1261 = property on="Confocal Image" class="Bool (strict)"("Val(Sgnl)"=TRUE ("Value (Signaling)")) -> ()  [unwired: 2 in, 2 out]
          }
          frame #5 {
            n1262 = Wait (ms)(milliseconds to wait=u32 2000) -> ()  [unwired: 1 out]
          }
          frame #6 {
            n1263 = while {
              stop <- w1953 stop-if-true
              n1264 = local read "Saving..."() -> (w1954:bool)
              n1265 = Not(x=w1954) -> (.not. x?=w1953:bool)
            }
          }
          frame #7 {
            n1266 = property on="Flip Green Filter" class="Bool (strict)"("Val(Sgnl)"=TRUE ("Value (Signaling)")) -> ()  [unwired: 2 in, 2 out]
            n1267 = property on="Green Laser ON/Interlacing" class="Bool (strict)"("Val(Sgnl)"=w1958) -> ()  [unwired: 2 in, 2 out]
            n1268 = property on="Green laser mode" class="RadioBtnsControl (strict)"("Val(Sgnl)"=w1957) -> ()  [unwired: 2 in, 2 out]
          }
          frame #8 {
            n1269 = property on="Green FB On/Off" class="Bool (strict)"("Val(Sgnl)"=w1959) -> ()  [unwired: 2 in, 2 out]
          }
        }
      }
      event "Stop All": Value Change {
        n1270 = event-data() -> ()  [unwired: 1 in, 5 out]
        n1271 = local read "Stop All"() -> (w1960:bool)
      }
    }
    n1272 = node-c288() -> ()  [unwired: 1 in, 1 out]
  }
  n1273 = node-c288() -> (w104:T25)  [unwired: 4 out]
  n1274 = timed-loop "Mouse control: trap position (AOM deflection), set confocal spot from image" {
    tunnel: [w1962] -> w64
    tunnel: w55 -> [w1961]
    timing: w104 -> [_]
    timing-out: [_] -> w103
    stop <- w1962 stop-if-true
    n1275 = node-c288() -> ()  [unwired: 2 out]
    n1276 = event shown="[0] \"Pane\": Mouse Down" {
      selector: _ -> [_ _]
      dyn-events: _ -> [_ _]
      timeout: _ -> [_ _]
      tunnel: w1961 -> [w1965 _]
      event Mouse Down {
        n1277 = event-data() -> ("Time"=w1967:u32, "Coords"=w1966:T8, "Button"=w1968:u16)  [unwired: 6 out]
        n1278 = case shown="1" w1968 {
          tunnel: w1967 -> [_ _ w2071]
          tunnel: w1966 -> [_ w2005 w2069]
          tunnel: w1965 -> [_ _ w2067]
          frame 0, Default {
          }
          frame 1 {
            n1279 = property on="APD 2" class="ImageControl"() -> ("Displayed Image Position"=w1975:cluster{"Left":i32, "Top":i32})  [unwired: 2 in, 2 out]
            n1280 = property on="APD 1" class="ImageControl"() -> ("Displayed Image Position"=w2004:cluster{"Left":i32, "Top":i32})  [unwired: 2 in, 2 out]
            n1281 = property on="Detection Laser X" class="ImageControl"() -> ("Displayed Image Position"=w2001:cluster{"Left":i32, "Top":i32})  [unwired: 2 in, 2 out]
            n1282 = property on="Detection Laser Y" class="ImageControl"() -> ("Displayed Image Position"=w2000:cluster{"Left":i32, "Top":i32})  [unwired: 2 in, 2 out]
            n1283 = property on="APD 2" class="ImageControl"() -> ("Displayed Image Size"=w1974:cluster{"Width":u32, "Height":u32})  [unwired: 2 in, 2 out]
            n1284 = property on="APD 1" class="ImageControl"() -> ("Displayed Image Size"=w2002:cluster{"Width":u32, "Height":u32})  [unwired: 2 in, 2 out]
            n1285 = property on="Detection Laser X" class="ImageControl"() -> ("Displayed Image Size"=w2003:cluster{"Width":u32, "Height":u32})  [unwired: 2 in, 2 out]
            n1286 = property on="Detection Laser Y" class="ImageControl"() -> ("Displayed Image Size"=w1999:cluster{"Width":u32, "Height":u32})  [unwired: 2 in, 2 out]
            n1287 = Unbundle By Name(w1974) -> ("Width"=w1971:u32, "Height"=w1970:u32)
            n1288 = Unbundle By Name(w1975) -> ("Left"=w1973:i32, "Top"=w1972:i32)
            n1289 = Unbundle By Name(w2002) -> ("Width"=w1996:u32, "Height"=w1995:u32)
            n1290 = Unbundle By Name(w2003) -> ("Width"=w1992:u32, "Height"=w1991:u32)
            n1291 = Unbundle By Name(w1999) -> ("Width"=w1988:u32, "Height"=w1987:u32)
            n1292 = Unbundle By Name(w2004) -> ("Left"=w1998:i32, "Top"=w1997:i32)
            n1293 = Unbundle By Name(w2001) -> ("Left"=w1994:i32, "Top"=w1993:i32)
            n1294 = Unbundle By Name(w2000) -> ("Left"=w1990:i32, "Top"=w1989:i32)
            n1295 = Bundle("Left"=w1973, "Top"=w1972, "Width"=w1971, "Height"=w1970) -> (w1969:T34)  [unwired: 1 in]
            n1296 = Bundle("Left"=w1998, "Top"=w1997, "Width"=w1996, "Height"=w1995) -> (w1986:T34)  [unwired: 1 in]
            n1297 = Bundle("Left"=w1994, "Top"=w1993, "Width"=w1992, "Height"=w1991) -> (w1985:T34)  [unwired: 1 in]
            n1298 = Bundle("Left"=w1990, "Top"=w1989, "Width"=w1988, "Height"=w1987) -> (w1984:T34)  [unwired: 1 in]
            n1299 = Build Cluster Array(w1969, w1986, w1985, w1984) -> (w1983:T35)
            n1300 = for {
              tunnel: w2005 -> [w2016]
              tunnel: w1983 -> [w2017] mode=indexing
              shift-right: [w2014] -> w1981
              shift-left: TRUE -> [w2015]
              shift-right: [w2013] -> w1979
              shift-left: _ -> [w2009]
              shift-right: [w2012] -> w1978
              shift-left: _ -> [w2008]
              shift-right: [w2011] -> w1977
              shift-left: _ -> [w2007]
              shift-right: [w2010] -> w1976
              shift-left: _ -> [w2006]
              n1301 = case shown="True" w2015 {
                selector: w2015 -> [w2022 _]
                tunnel: w2017 -> [_ w2031]
                tunnel: w2016 -> [_ w2029]
                tunnel: [w2022 w2027] -> w2014
                tunnel: [w2021 w2026] -> w2013
                tunnel: [w2020 w2025] -> w2012
                tunnel: [w2019 w2024] -> w2011
                tunnel: [w2018 w2023] -> w2010
                tunnel: w2009 -> [w2021 _]
                tunnel: w2008 -> [w2020 _]
                tunnel: w2007 -> [w2019 _]
                tunnel: w2006 -> [w2018 _]
                frame False {
                }
                frame True {
                  n1302 = Unbundle(w2031) -> (w2030:T34)
                  n1303 = call "isclickinwindow.vi"("Image Param"=w2030, "Point32"=w2029) -> ("Y px"=w2023:i32, "Height"=w2024:i32, "X px"=w2025:i32, "Width"=w2026:i32, "In image?"=w2028:bool)  [unwired: 1 in]
                  n1304 = Not(x=w2028) -> (.not. x?=w2027:bool)
                }
              }
            }
            n1305 = Not(x=w1981) -> (.not. x?=w1980:bool)
            n1306 = case shown="True" w1980 {
              tunnel: w1978 -> [_ w2044]
              tunnel: w1976 -> [_ w2043]
              tunnel: w1979 -> [_ w2042]
              tunnel: w1977 -> [_ w2041]
              frame False {
              }
              frame True {
                w2037 = FALSE ("Get Point")
                n1307 = local read "Scan lines (y)"() -> (w2046:u64)
                n1308 = local read "Actual MCL Inc (V)"() -> (w2038:dbl)
                n1309 = local read "Scan steps (MCL)"() -> (w2045:u64)
                n1310 = Divide "Y Pix/step"(x=w2041, y=w2046) -> (x/y=w2053:dbl)
                n1311 = Divide "Y V/pix"(x=w2038, y=w2053) -> (x/y=w2052:dbl)
                n1312 = Divide "Y half step offset"(x=w2038, y=2.0) -> (x/y=w2054:dbl)
                n1313 = Divide "X pix/step"(x=w2042, y=w2045) -> (x/y=w2051:dbl)
                n1314 = Negate(x=w2054) -> (-x=w2055:dbl)
                n1315 = local read "Initial Y"() -> (w2061:dbl)
                n1316 = Multiply(x=w2043, y=w2052) -> (x*y=w2062:dbl)
                n1317 = Divide "X half step offset"(x=w2038, y=2.0) -> (x/y=w2048:dbl)
                n1318 = Divide "X V/pix"(x=w2038, y=w2051) -> (x/y=w2050:dbl)
                n1319 = Multiply(x=w2038, y=w2045) -> (x*y=w2057:dbl)
                n1320 = Compound Arithmetic op=ADD(w2055, w2062, w2061) -> (w2039:dbl)
                "Pointer Y (V)" <- w2039
                n1321 = Multiply(x=w2050, y=w2044) -> (x*y=w2059:dbl)
                n1322 = Negate(x=w2048) -> (-x=w2047:dbl)
                n1323 = local read "Initial X"() -> (w2060:dbl)
                n1324 = Negate(x=w2059) -> (-x=w2058:dbl)
                n1325 = Compound Arithmetic op=ADD(w2047, w2057, w2060, w2058) -> (w2040:dbl)
                "Pointer X (V)" <- w2040
                n1326 = Or(x="Set X Only", y="Set Confocal Spot (X-Y)") -> (x .or. y?=w2033:bool)
                n1327 = Or(x="Set Confocal Spot (X-Y)", y="Set Y Only") -> (x .or. y?=w2032:bool)
                n1328 = case shown="True" w2033 {
                  tunnel: w2040 -> [_ w2063]
                  frame False {
                  }
                  frame True {
                    n1329 = property on="AO2" class="Slide (strict)"("Val(Sgnl)"=w2063) -> ()  [unwired: 2 in, 2 out]
                  }
                }
                n1330 = case shown="True" w2032 {
                  tunnel: w2039 -> [_ w2064]
                  frame False {
                  }
                  frame True {
                    n1331 = property on="AO1" class="Slide (strict)"("Val(Sgnl)"=w2064) -> ()  [unwired: 2 in, 2 out]
                  }
                }
                n1332 = local write "Set Confocal Spot (X-Y)"(w2037) -> ()
                n1333 = local write "Set X Only"(w2037) -> ()
                n1334 = local write "Set Y Only"(w2037) -> ()
              }
            }
          }
          frame 3 {
            n1335 = local read "BD 2 Frequency 1 (MHz)"() -> (w2065:dbl)
            n1336 = local read "BD 1 Frequency 1 (MHz)"() -> (w2066:dbl)
            n1337 = local write "Manipulating Trap"(TRUE ("Manipulating Trap")) -> ()
            n1338 = local write "Coords"(T8 {"Horizontal"=0, "Vertical"=0} ("Coords")) -> ()
            n1339 = while {
              tunnel: w2071 -> [w2076]
              tunnel: w2069 -> [w2075]
              tunnel: w2067 -> [w2074]
              tunnel: w2066 -> [w2073]
              tunnel: w2065 -> [w2072]
              stop <- w2077 stop-if-true
              n1340 = event shown="[0] \"Pane\": Mouse Move" {
                selector: _ -> [_ _]
                dyn-events: _ -> [_ _]
                timeout: _ -> [_ _]
                tunnel: ["Force Manip Abort" w2141] -> w2077
                tunnel: w2076 -> [w2084 _]
                tunnel: w2075 -> [w2082 _]
                tunnel: w2074 -> [w2081 _]
                tunnel: w2073 -> [w2080 _]
                tunnel: w2072 -> [w2079 _]
                event Mouse Move {
                  n1341 = event-data() -> ("Time"=w2085:u32, "Coords"=w2086:T8)  [unwired: 3 out]
                  n1342 = Less?(x=w2085, y=w2084) -> (x < y?=w2083:bool)
                  n1343 = case "Makes sure old motion events prior to mouse click aren't used" shown="False" w2083 {
                    tunnel: w2086 -> [w2128 _]
                    tunnel: w2082 -> [w2129 _]
                    tunnel: w2081 -> [w2106 _]
                    tunnel: w2080 -> [w2102 _]
                    tunnel: w2079 -> [w2101 _]
                    frame False {
                      n1344 = Subtract(x=w2128, y=w2129) -> (x-y=w2127:T8)
                      "Coords" <- w2127
                      n1345 = local read "Y RF Frequency Limits (MHz)"() -> (w2087:T16)
                      n1346 = To Double Precision Float(number=w2127) -> (double precision float=w2126:cluster{"Horizontal":dbl, "Vertical":dbl})
                      n1347 = Multiply(x=cluster{"Horizontal":dbl, "Vertical":dbl} {"Horizontal"=-1.0, "Vertical"=1.0}, y="Manipulation Scaling") -> (x*y=w2122:cluster{"Horizontal":dbl, "Vertical":dbl})
                      n1348 = local read "X RF Frequency Limits (MHz)"() -> (w2088:T16)
                      n1349 = Multiply(x=w2126, y=w2122) -> (x*y=w2124:cluster{"Horizontal":dbl, "Vertical":dbl})
                      n1350 = Unbundle By Name(w2124) -> ("Horizontal"=w2119:dbl, "Vertical"=w2123:dbl)
                      n1351 = Unbundle By Name(w2087) -> ("Maximum"=w2090:dbl, "Minimum"=w2089:dbl)
                      n1352 = Boolean To (0,1)(Boolean="Manip. X?") -> (0, 1=w2117:i16)
                      n1353 = Boolean To (0,1)(Boolean="Manip. Y?") -> (0, 1=w2114:i16)
                      n1354 = local read "BD 1 Frequency 2 (MHz)"() -> (w2104:dbl)
                      n1355 = Multiply(x=w2123, y=w2114) -> (x*y=w2116:dbl)
                      n1356 = Multiply(x=w2117, y=w2119) -> (x*y=w2120:dbl)
                      n1357 = local read "BD 2 Frequency 2 (MHz)"() -> (w2103:dbl)
                      n1358 = Unbundle By Name(w2088) -> ("Maximum"=w2092:dbl, "Minimum"=w2091:dbl)
                      n1359 = Add(x=w2101, y=w2116) -> (x+y=w2094:dbl)
                      n1360 = Add(x=w2102, y=w2120) -> (x+y=w2096:dbl)
                      n1361 = In Range and Coerce(upper limit=w2092, x=w2096, lower limit=w2091) -> (coerced(x)=w2095:dbl)  [unwired: 1 out]
                      n1362 = In Range and Coerce(upper limit=w2090, x=w2094, lower limit=w2089) -> (coerced(x)=w2093:dbl)  [unwired: 1 out]
                      n1363 = Subtract(x=w2095, y=w2104) -> (x-y=w2113:dbl)
                      n1364 = Subtract(x=w2093, y=w2103) -> (x-y=w2112:dbl)
                      n1365 = Square(x=w2113) -> (x^2=w2111:dbl)
                      n1366 = Square(x=w2112) -> (x^2=w2110:dbl)
                      n1367 = Add(x=w2111, y=w2110) -> (x+y=w2109:dbl)
                      n1368 = Square Root(x=w2109) -> (sqrt(x)=w2105:dbl)
                      n1369 = In Range and Coerce(upper limit="Limit Max (MHz)", x=w2105, lower limit="Limit Min (MHz)") -> (In Range?=w2098:bool)  [unwired: 1 out]
